vi "Read PWM-Ratio-URLs.vi"(8 "error in (no error)":errorcluster, 11 "BNT_ULx-MCSV-DOPWM in":refnum<class "BNT_ULx-MCSV-DOPWM.lvclass">) -> (0 "error out":errorcluster, 2 "PWM-Ratio-URLs":string[](array[string]), 3 "BNT_ULx-MCSV-DOPWM out":refnum<class "BNT_ULx-MCSV-DOPWM.lvclass">)   [LabVIEW 2021, in "BNT_ULx.lvlib" / "BNT_ULx-MCSV-DOPWM.lvclass"]
uses:
  BNT_ULx-MCSV-DOPWM.lvclass
  BNT_ULx-MCSV-DOPWM.lvclass/BNT_ULx-MCSV-DOPWM.ctl
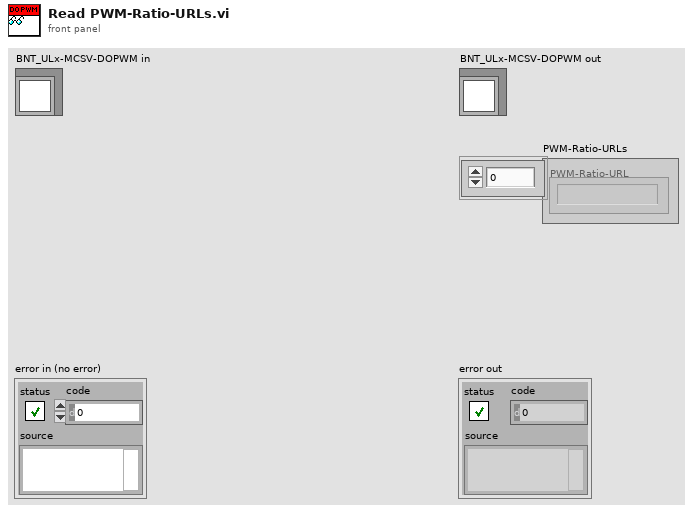
[diagram p1: front panel]
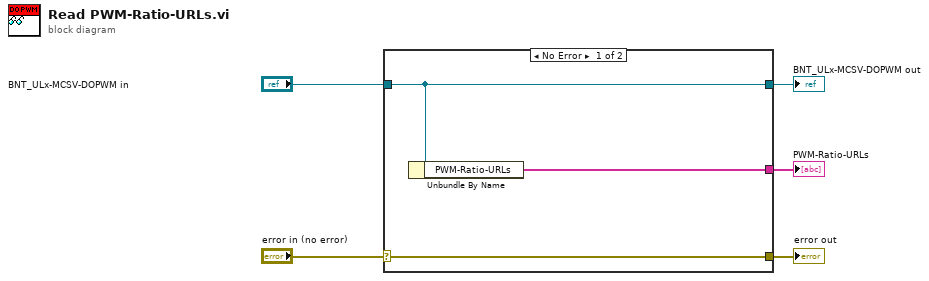
[diagram p0: block diagram]
diagram:
  n1 = case shown="No Error" "error in (no error)" {
    selector: "error in (no error)" -> [w8 w9]
    tunnel: [w8 w9] -> w4
    tunnel: [w7 w10] -> w2
    tunnel: "BNT_ULx-MCSV-DOPWM in" -> [w7 w10]
    tunnel: [w6 _] -> w1
    frame No Error {
      n2 = Unbundle By Name(w7) -> ("PWM-Ratio-URLs"=w6:string[])
    }
    frame Error {
    }
  }
  "error out" <- w4
  "BNT_ULx-MCSV-DOPWM out" <- w2
  "PWM-Ratio-URLs" <- w1
